vi "Checkers Settings.vi"() -> ()   [LabVIEW 2016]
uses:
  Game Info Global Variable.vi
panel:
  in  "P2 Blue Text Color:":i32
  in  "P2 Green Text Color:":i32
  in  "P2 Red Text Color:":i32
  in  "P2 Blue Color:":i32
  in  "P2 Green Color:":i32
  in  "P2 Red Color:":i32
  in  "P1 Blue Text Color:":i32
  in  "P1 Green Text Color:":i32
  in  "P1 Red Text Color:":i32
  in  "P1 Blue Color:":i32
  in  "P1 Green Color:":i32
  in  "P1 Red Color:":i32
  in  "Blue:":string="255"
  in  "Green:":string="255"
  in  "Red:":string="255"
  in  "Blue:":string="0"
  in  "Green:":string="0"
  in  "Red:":string="0"
  in  "Main Menu":bool
  in  "Apply Changes":bool
  out "new picture 4":picture
  out "new picture 2":picture
  out "new picture":picture
  out "new picture 3":picture
  out "King:":picture
  out "Piece:":picture
  # "SETTINGS:"
  # "Player 1 Piece/King Color:"
  # "Turn Marker:"
  # "Piece:"
  # "King:"
  # "Player 1 King Text Color:"
  # "Player 2 Piece/King Color:"
  # "Piece:"
  # "King:"
  # "Turn Marker:"
  # "Player 2 King Text Color:"
  # "Board Square Color 1:"
  # "Board Square 1:"
  # "Board Square 1:"
  # "Board Square Color 2:"
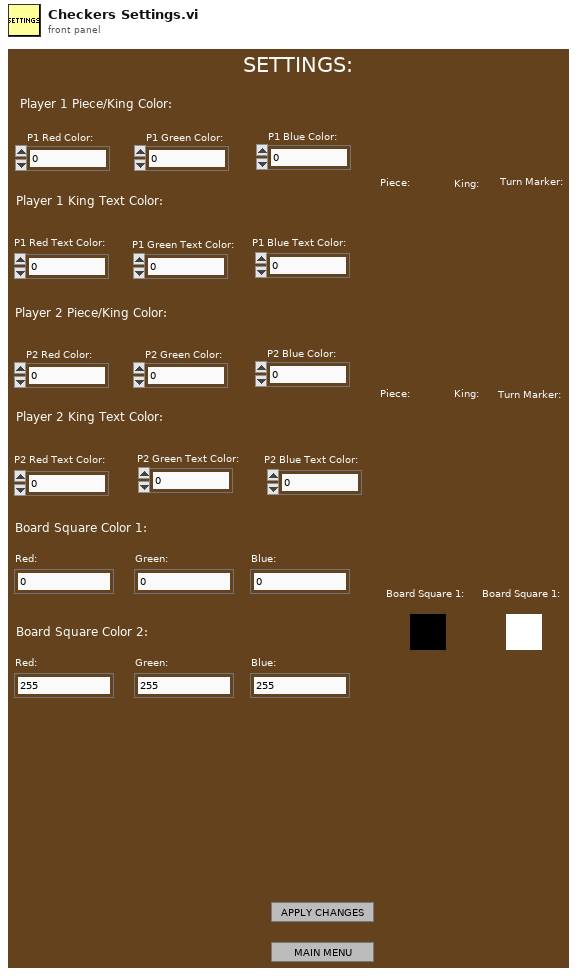
[diagram p1: front panel]
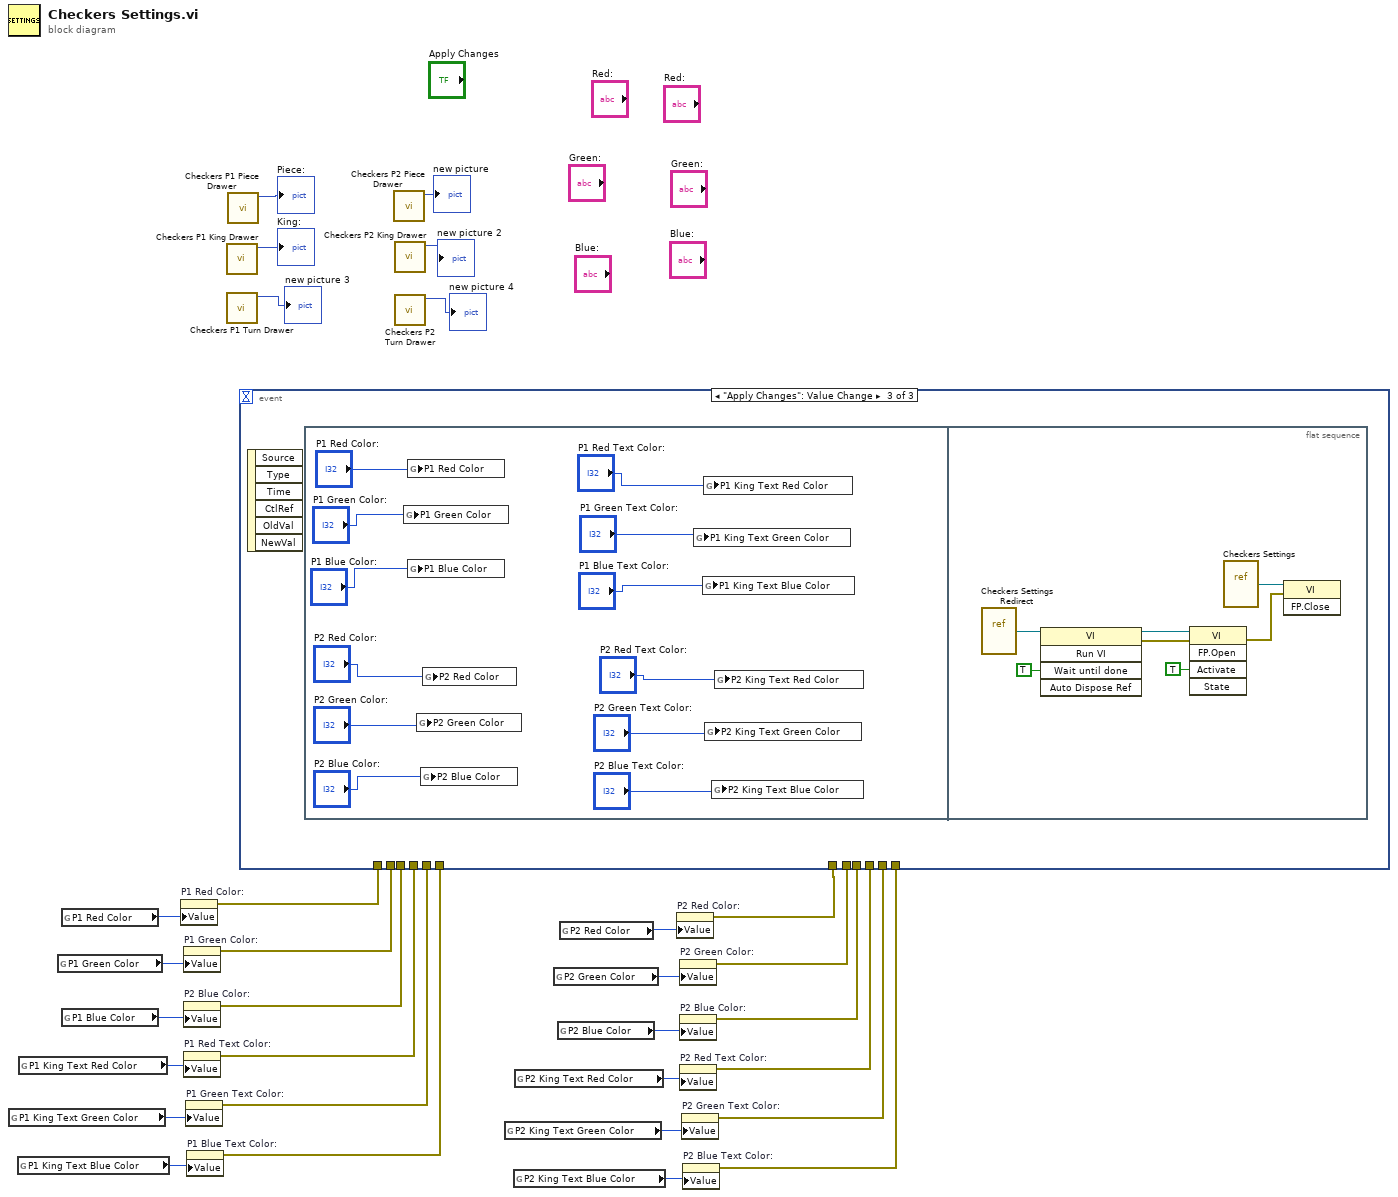
[diagram p0: block diagram]
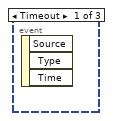
[diagram p2: hidden frame]
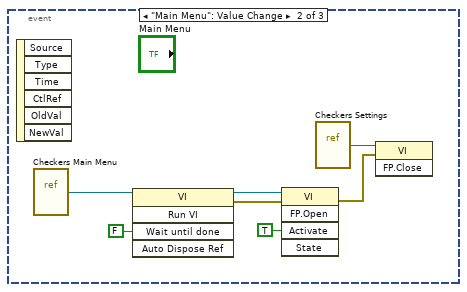
[diagram p3: hidden frame]
diagram:
  n1 = global read "Game Info Global Variable.vi" "P1 King Text Green Color"() -> (w17:i32)
  n2 = global read "Game Info Global Variable.vi" "P1 King Text Blue Color"() -> (w16:i32)
  n3 = global read "Game Info Global Variable.vi" "P1 King Text Red Color"() -> (w18:i32)
  n4 = global read "Game Info Global Variable.vi" "P1 Green Color"() -> (w22:i32)
  n5 = global read "Game Info Global Variable.vi" "P1 Red Color"() -> (w24:i32)
  n6 = global read "Game Info Global Variable.vi" "P1 Blue Color"() -> (w20:i32)
  n7 = property on="P1 Red Color:" class="DigNum (strict)"("Value"=w24) -> (error out=w23:errorcluster)  [unwired: 2 in, 1 out]
  n8 = property on="P1 Green Color:" class="DigNum (strict)"("Value"=w22) -> (error out=w21:errorcluster)  [unwired: 2 in, 1 out]
  n9 = property on="P2 Blue Color:" class="DigNum (strict)"("Value"=w20) -> (error out=w19:errorcluster)  [unwired: 2 in, 1 out]
  n10 = property on="P1 Red Text Color:" class="DigNum (strict)"("Value"=w18) -> (error out=w15:errorcluster)  [unwired: 2 in, 1 out]
  n11 = property on="P1 Green Text Color:" class="DigNum (strict)"("Value"=w17) -> (error out=w14:errorcluster)  [unwired: 2 in, 1 out]
  n12 = property on="P1 Blue Text Color:" class="DigNum (strict)"("Value"=w16) -> (error out=w13:errorcluster)  [unwired: 2 in, 1 out]
  n13 = call "Checkers P1 King Drawer.vi"() -> ("new picture"=→"King:":picture)  [unwired: 11 in]
  n14 = call "Checkers P1 Turn Drawer.vi"() -> ("new picture"=→"new picture 3":picture)  [unwired: 11 in]
  n15 = call "Checkers P1 Piece Drawer.vi"() -> ("new picture"=→"Piece:":picture)  [unwired: 11 in]
  n16 = call "Checkers P2 Piece Drawer.vi"() -> ("new picture"=→"new picture":picture)  [unwired: 11 in]
  n17 = call "Checkers P2 King Drawer.vi"() -> ("new picture"=→"new picture 2":picture)  [unwired: 11 in]
  n18 = call "Checkers P2 Turn Drawer.vi"() -> ("new picture"=→"new picture 4":picture)  [unwired: 11 in]
  n19 = global read "Game Info Global Variable.vi" "P2 King Text Green Color"() -> (w11:i32)
  n20 = global read "Game Info Global Variable.vi" "P2 King Text Blue Color"() -> (w12:i32)
  n21 = global read "Game Info Global Variable.vi" "P2 King Text Red Color"() -> (w10:i32)
  n22 = global read "Game Info Global Variable.vi" "P2 Green Color"() -> (w8:i32)
  n23 = global read "Game Info Global Variable.vi" "P2 Blue Color"() -> (w9:i32)
  n24 = global read "Game Info Global Variable.vi" "P2 Red Color"() -> (w7:i32)
  n25 = property on="P2 Red Color:" class="DigNum (strict)"("Value"=w7) -> (error out=w6:errorcluster)  [unwired: 2 in, 1 out]
  n26 = property on="P2 Green Color:" class="DigNum (strict)"("Value"=w8) -> (error out=w5:errorcluster)  [unwired: 2 in, 1 out]
  n27 = property on="P2 Blue Color:" class="DigNum (strict)"("Value"=w9) -> (error out=w4:errorcluster)  [unwired: 2 in, 1 out]
  n28 = property on="P2 Red Text Color:" class="DigNum (strict)"("Value"=w10) -> (error out=w3:errorcluster)  [unwired: 2 in, 1 out]
  n29 = property on="P2 Green Text Color:" class="DigNum (strict)"("Value"=w11) -> (error out=w2:errorcluster)  [unwired: 2 in, 1 out]
  n30 = property on="P2 Blue Text Color:" class="DigNum (strict)"("Value"=w12) -> (error out=w1:errorcluster)  [unwired: 2 in, 1 out]
  n31 = event shown="[2] \"Apply Changes\": Value Change" {
    selector: _ -> [_ _ _]
    dyn-events: _ -> [_ _ _]
    timeout: _ -> [_ _ _]
    tunnel: w23 -> [_ _ _]
    tunnel: w21 -> [_ _ _]
    tunnel: w19 -> [_ _ _]
    tunnel: w15 -> [_ _ _]
    tunnel: w14 -> [_ _ _]
    tunnel: w13 -> [_ _ _]
    tunnel: w6 -> [_ _ _]
    tunnel: w5 -> [_ _ _]
    tunnel: w4 -> [_ _ _]
    tunnel: w3 -> [_ _ _]
    tunnel: w2 -> [_ _ _]
    tunnel: w1 -> [_ _ _]
    event Timeout {
      n32 = event-data() -> ()  [unwired: 1 in, 3 out]
    }
    event "Main Menu": Value Change {
      n33 = event-data() -> ()  [unwired: 1 in, 6 out]
      n34 = vi-ref "Checkers Main Menu.vi"() -> (w37:refnum<vi>)
      n35 = invoke class="VI" method="Run VI"(reference=w37, "Wait until done"=FALSE ("Wait Until Done")) -> (reference out=w36:refnum<vi>, error out=w35:errorcluster)  [unwired: 3 in, 3 out]
      n36 = invoke class="VI" method="FP.Open"(reference=w36, error in=w35, "Activate"=TRUE ("Activate?")) -> (error out=w31:errorcluster)  [unwired: 2 in, 4 out]
      n37 = vi-ref "Checkers Settings.vi"() -> (w32:refnum<vi>)
      n38 = invoke class="VI" method="FP.Close"(reference=w32, error in=w31) -> ()  [unwired: 1 in, 3 out]
    }
    event "Apply Changes": Value Change {
      n39 = event-data() -> ()  [unwired: 1 in, 6 out]
      n40 = flat-sequence {
        frame #0 {
          n41 = global write "Game Info Global Variable.vi" "P1 Green Color"("P1 Green Color:") -> ()
          n42 = global write "Game Info Global Variable.vi" "P1 Red Color"("P1 Red Color:") -> ()
          n43 = global write "Game Info Global Variable.vi" "P1 Blue Color"("P1 Blue Color:") -> ()
          n44 = global write "Game Info Global Variable.vi" "P2 Green Color"("P2 Green Color:") -> ()
          n45 = global write "Game Info Global Variable.vi" "P2 Blue Color"("P2 Blue Color:") -> ()
          n46 = global write "Game Info Global Variable.vi" "P2 Red Color"("P2 Red Color:") -> ()
          n47 = global write "Game Info Global Variable.vi" "P1 King Text Green Color"("P1 Green Text Color:") -> ()
          n48 = global write "Game Info Global Variable.vi" "P1 King Text Blue Color"("P1 Blue Text Color:") -> ()
          n49 = global write "Game Info Global Variable.vi" "P1 King Text Red Color"("P1 Red Text Color:") -> ()
          n50 = global write "Game Info Global Variable.vi" "P2 King Text Green Color"("P2 Green Text Color:") -> ()
          n51 = global write "Game Info Global Variable.vi" "P2 King Text Blue Color"("P2 Blue Text Color:") -> ()
          n52 = global write "Game Info Global Variable.vi" "P2 King Text Red Color"("P2 Red Text Color:") -> ()
        }
        frame #1 {
          n53 = vi-ref "Checkers Settings Redirect.vi"() -> (w56:refnum<vi>)
          n54 = invoke class="VI" method="Run VI"(reference=w56, "Wait until done"=TRUE ("Wait Until Done")) -> (reference out=w55:refnum<vi>, error out=w54:errorcluster)  [unwired: 3 in, 3 out]
          n55 = invoke class="VI" method="FP.Open"(reference=w55, error in=w54, "Activate"=TRUE ("Activate?")) -> (error out=w51:errorcluster)  [unwired: 2 in, 4 out]
          n56 = vi-ref "Checkers Settings.vi"() -> (w50:refnum<vi>)
          n57 = invoke class="VI" method="FP.Close"(reference=w50, error in=w51) -> ()  [unwired: 1 in, 3 out]
        }
      }
    }
  }
